vi "DeployMe.vi"() -> ()   [LabVIEW 2011]
uses:
  C:/Dev/tsdev/Dev/5.1/App/TestStand/Components/Tools/MigrationUtility/NationalInstruments.TestStand.Utility.dll
  Dev/tsdev/Dev/5.1/App/TestStand/Components/Tools/MigrationUtility/NationalInstruments.TestStand.Utility.dll
panel:
  out "Exists":bool
  out "error out":errorcluster
  in  "error in (no error)":errorcluster
  in  "Path":path
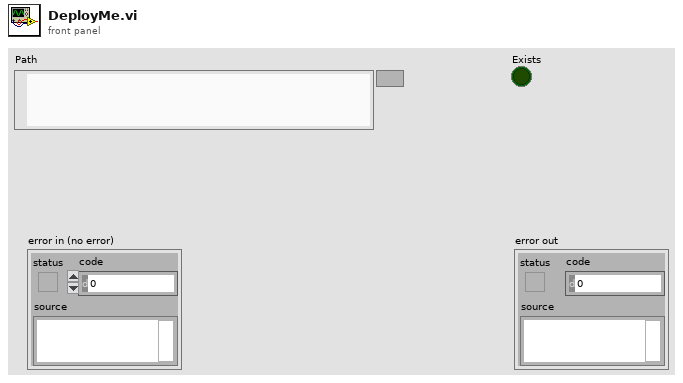
[diagram p1: front panel]
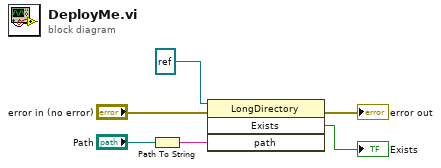
[diagram p0: block diagram]
diagram:
  n1 = Path To String(path="Path") -> (string=w1:string)
  n2 = invoke class="LongDirectory" method="Exists"(reference=refnum<k24> refnum, error in="error in (no error)", "path"=w1) -> (error out=→"error out":errorcluster, "Exists"=→"Exists":bool)  [unwired: 1 in, 2 out]
